vi "GetControlBackgroundColor.vi"(7 "VI Interpreter in":refnum<class "VI Interpreter.lvclass">, 8 "error in":errorcluster, 11 "Control in":refnum<class "Control.lvclass">) -> (0 "error out":errorcluster, 3 "Control out":refnum<class "Control.lvclass">, 4 "BG color":u32(colorbox), 5 "VI Interpreter out":refnum<class "VI Interpreter.lvclass">)   [LabVIEW 2014, in "PythonConverter_GUI.lvclass"]
uses:
  PythonConverter_GUI.lvclass
  VI Interpreter/Classes/Control/Control.lvclass
  VI Interpreter/Classes/VI Interpreter/VI Interpreter.lvclass
  VI Interpreter/Classes/Generic/Generic.lvclass/Generic.ctl
  VI Interpreter/Classes/Tab/Tab.lvclass/Tab.ctl
  VI Interpreter/Classes/PageSelector/PageSelector.lvclass/PageSelector.ctl
  VI Interpreter/Classes/Page/Page.lvclass/Page.ctl
  VI Interpreter/Classes/Cluster/Cluster.lvclass/Cluster.ctl
  VI Interpreter/Classes/Pane/Pane.lvclass/Pane.ctl
  VI Interpreter/Classes/Generic/Generic.lvclass
  VI Interpreter/Classes/Tab/Tab.lvclass
  VI Interpreter/Classes/PageSelector/PageSelector.lvclass
  VI Interpreter/Classes/Page/Page.lvclass
  VI Interpreter/Classes/Pane/Pane.lvclass
  VI Interpreter/Classes/Cluster/Cluster.lvclass
  VI Interpreter/Classes/Array/Array.lvclass
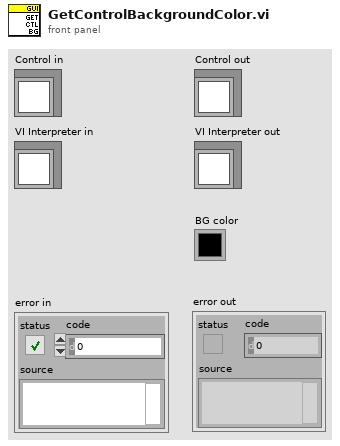
[diagram p1: front panel]
types:
  T1 = typedef "TabStyleTD.ctl" = enum16{"system", "modern", "classic"}
  T2 = typedef "LVForegroundBackgroundColorsTypeDef.ctl" = cluster{"Foreground Color":u32, "Background Color":u32}
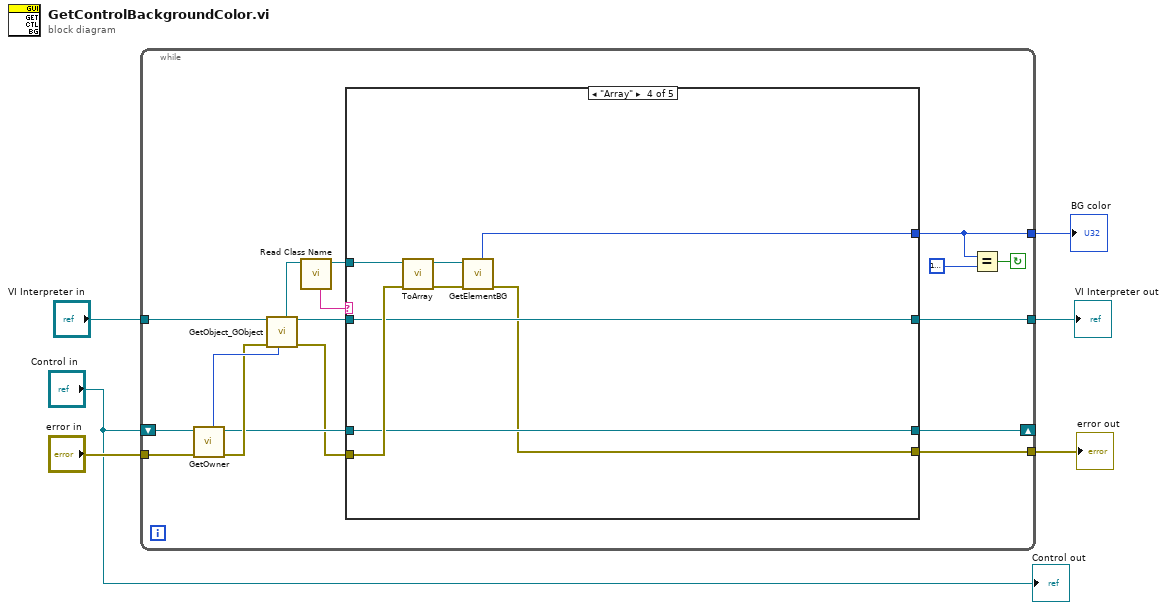
[diagram p0: block diagram]
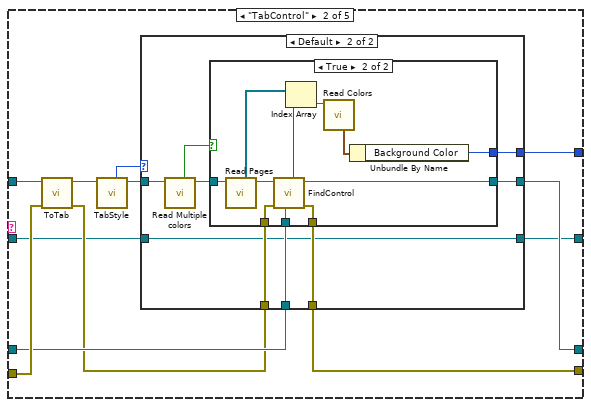
[diagram p3: hidden frame]
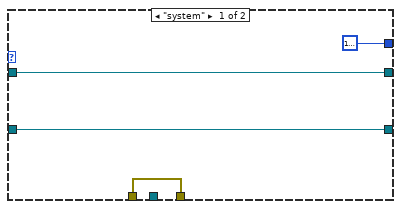
[diagram p4: hidden frame]
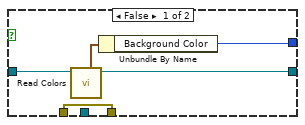
[diagram p5: hidden frame]
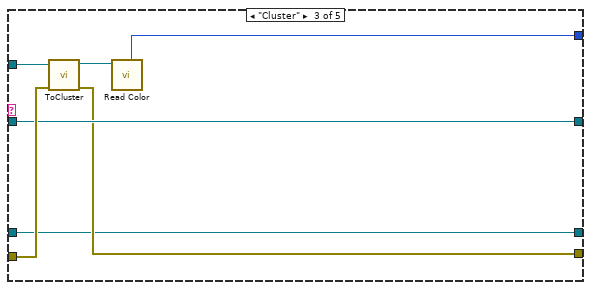
[diagram p6: hidden frame]
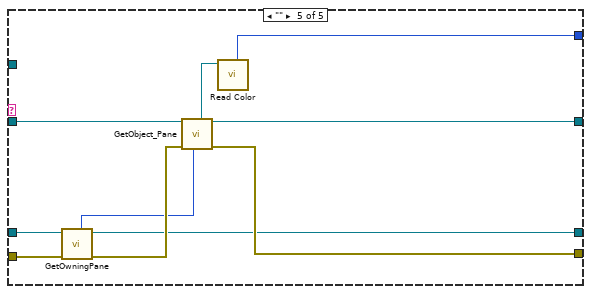
[diagram p7: hidden frame]
diagram:
  n1 = while {
    tunnel: "error in" -> [w23]
    tunnel: "VI Interpreter in" -> [w21]
    tunnel: [w9] -> w4
    tunnel: [w14] -> w3
    tunnel: [w12] -> w2
    shift-right: [w10] -> _
    shift-left: "Control in" -> [w22]
    stop <- w7 continue-if-true
    n2 = call-dynamic "GetOwner.vi"("error in"=w23, "Control in"=w22) -> ("error out"=w19:errorcluster, "Control out"=w13:refnum<class "Control.lvclass">, "Owner"=w20:i32)  [unwired: 5 in]
    n3 = call "GetObject_GObject.vi"("UID"=w20, "error in"=w19, "VI Interpreter in"=w21) -> ("error out"=w11:errorcluster, "VI Interpreter out"=w15:refnum<class "VI Interpreter.lvclass">, "GObject"=w18:refnum<class "GObject.lvclass">)  [unwired: 3 in, 1 out]
    n4 = call "Read Class Name.vi"("Generic in"=w18) -> ("Generic out"=w16:refnum<class "GObject.lvclass">, "Class Name"=w17:string)  [unwired: 7 in]
    n5 = case shown="\"Array\"" w17 {
      tunnel: w16 -> [_ w38 w74 w82 _]
      tunnel: [_ w34 w70 w78 w92] -> w9
      tunnel: w15 -> [w26 w28 w72 w77 w89]
      tunnel: [w26 w29 w72 w77 w88] -> w14
      tunnel: w13 -> [w24 w36 w68 w76 w90]
      tunnel: [w25 w35 w69 w75 w86] -> w12
      tunnel: w11 -> [w25 w37 w73 w81 w91]
      tunnel: [w24 w32 w68 w76 w83] -> w10
      frame Default {
      }
      frame "TabControl" {
        n6 = call "ToTab.vi"("error in"=w37, "Generic in"=w38) -> ("error out"=w33:errorcluster, "Tab out"=w31:refnum<class "Tab.lvclass">)  [unwired: 8 in]
        n7 = call "TabStyle.vi"("Tab in"=w31) -> ("Tab out"=w30:refnum<class "Tab.lvclass">, "Tab style"=w27:T1)  [unwired: 7 in]
        n8 = case shown="Default" w27 {
          tunnel: w36 -> [_ w51]
          tunnel: [w39 w50] -> w35
          tunnel: [u32 16777226 w49] -> w34
          tunnel: w33 -> [w39 w46]
          tunnel: [w41 w45] -> w32
          tunnel: w30 -> [w41 w44]
          tunnel: [w42 w43] -> w29
          tunnel: w28 -> [w42 w43]
          frame "system" {
          }
          frame Default {
            n9 = call "Read Multiple colors.vi"("Tab in"=w44) -> ("Tab out"=w48:refnum<class "Tab.lvclass">, "Multiple colors"=w47:bool)  [unwired: 7 in]
            n10 = case shown="True" w47 {
              tunnel: w51 -> [_ w67]
              tunnel: [w55 w66] -> w50
              tunnel: [w53 w60] -> w49
              tunnel: w48 -> [w56 w59]
              tunnel: w46 -> [w55 w58]
              tunnel: [w52 w57] -> w45
              frame False {
                n11 = call "Read Colors.vi"("Tab in"=w56) -> ("Tab out"=w52:refnum<class "Tab.lvclass">, "Colors"=w54:T2)  [unwired: 7 in]
                n12 = Unbundle By Name(w54) -> ("Background Color"=w53:u32)
              }
              frame True {
                n13 = call "Read Pages.vi"("PageSelector in"=w59) -> ("PageSelector out"=w64:refnum<class "Tab.lvclass">, "Pages"=w65:refnum<class "Page.lvclass">[])  [unwired: 7 in]
                n14 = call "FindControl.vi"("Control in"=w67, "error in"=w58, "Tab in"=w64) -> ("error out"=w66:errorcluster, "Tab out"=w57:refnum<class "Tab.lvclass">, "Tab index"=w63:i32)  [unwired: 4 in]
                n15 = Index Array(array=w65, index=w63) -> (element=w62:refnum<class "Page.lvclass">)
                n16 = call "Read Colors.vi"("Page in"=w62) -> ("Colors"=w61:T2)  [unwired: 7 in, 1 out]
                n17 = Unbundle By Name(w61) -> ("Background Color"=w60:u32)
              }
            }
          }
        }
      }
      frame "Cluster" {
        n18 = call "ToCluster.vi"("error in"=w73, "Generic"=w74) -> ("error out"=w69:errorcluster, "Cluster out"=w71:refnum<class "Cluster.lvclass">)  [unwired: 8 in]
        n19 = call "Read Color.vi"("Cluster in"=w71) -> ("Color"=w70:u32)  [unwired: 7 in, 1 out]
      }
      frame "Array" {
        n20 = call "ToArray.vi"("error in"=w81, "Generic in"=w82) -> ("error out"=w79:errorcluster, "Array out"=w80:refnum<class "Array.lvclass">)  [unwired: 8 in]
        n21 = call "GetElementBG.vi"("error in"=w79, "Array in"=w80) -> ("error out"=w75:errorcluster, "Element BG"=w78:u32)  [unwired: 5 in, 1 out]
      }
      frame "" {
        n22 = call-dynamic "GetOwningPane.vi"("error in"=w91, "Control in"=w90) -> ("error out"=w87:errorcluster, "Control out"=w83:refnum<class "Control.lvclass">, "Owning Pane"=w84:i32)  [unwired: 5 in]
        n23 = call "GetObject_Pane.vi"("UID"=w84, "error in"=w87, "VI Interpreter in"=w89) -> ("error out"=w86:errorcluster, "VI Interpreter out"=w88:refnum<class "VI Interpreter.lvclass">, "pane"=w85:refnum<class "Pane.lvclass">)  [unwired: 3 in, 1 out]
        n24 = call "Read Color.vi"("Pane in"=w85) -> ("Color"=w92:u32)  [unwired: 7 in, 1 out]
      }
    }
    n25 = Equal?(x=w9, y=u32 16777216) -> (x = y?=w7:bool)
  }
  "error out" <- w2
  "BG color" <- w4
  "VI Interpreter out" <- w3
  "Control out" <- "Control in"
